vi "Set Connection ID.vi"(8 "error in (no error)":errorcluster, 10 "Connection ID":refnum<k5>, 11 "GenNet Protocol in":refnum<class "GenNet Protocol.lvclass">) -> (0 "error out":errorcluster, 3 "GenNet Protocol out":refnum<class "GenNet Protocol.lvclass">)   [LabVIEW 2020, in "hse-gennet.lvlib" / "GenNet Protocol.lvclass"]
doc: "____\nHAMPEL SOFTWARE ENGINEERING v3.8.0 (2023-12-18 14:41)"
uses:
  GenNet Protocol.lvclass
  GenNet Protocol.lvclass/GenNet Protocol.ctl
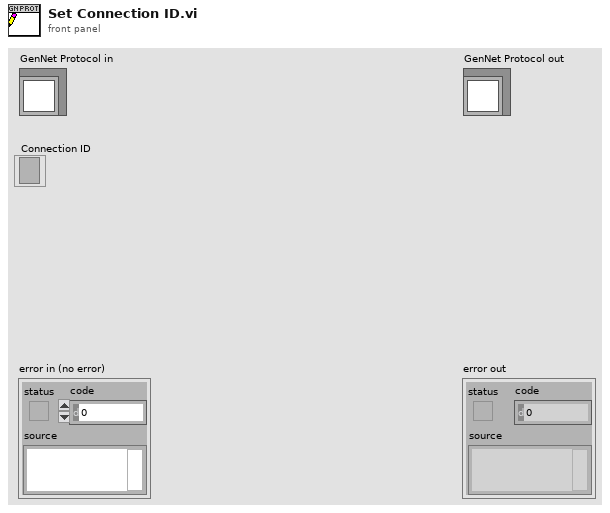
[diagram p1: front panel]
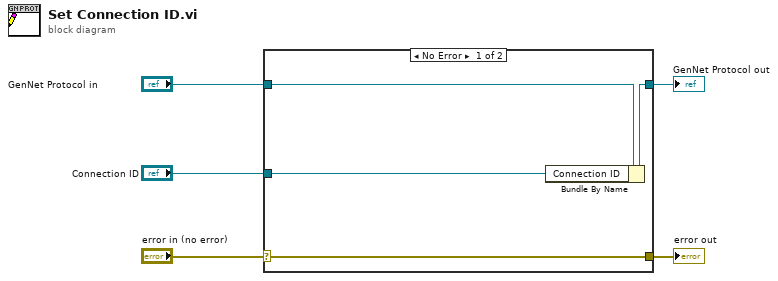
[diagram p0: block diagram]
diagram:
  n1 = case shown="No Error" "error in (no error)" {
    selector: "error in (no error)" -> [w9 w10]
    tunnel: [w9 w10] -> w4
    tunnel: [w7 w11] -> w2
    tunnel: "GenNet Protocol in" -> [w8 w11]
    tunnel: "Connection ID" -> [w6 _]
    frame No Error {
      n2 = Bundle By Name(cluster=w8, "Connection ID"=w6) -> (w7:refnum<class "GenNet Protocol.lvclass">)
    }
    frame Error {
    }
  }
  "error out" <- w4
  "GenNet Protocol out" <- w2
